vi "TDMS Write.vi"(7 "Channel Name":string, 8 "error in (no error)":errorcluster, 9 "Group Name":string, 10 "TDMS in":refnum<k34>, 11 "I32 in":refnum<class "I32.lvclass">) -> (0 "error out":errorcluster, 2 "TDMS Out":refnum<k34>)   [LabVIEW 2020, in "Data.lvlib" / "I32.lvclass"]
doc: "Write Generic Data to a TDMS file."
uses:
  I32.lvclass
  I32.lvclass/I32.ctl
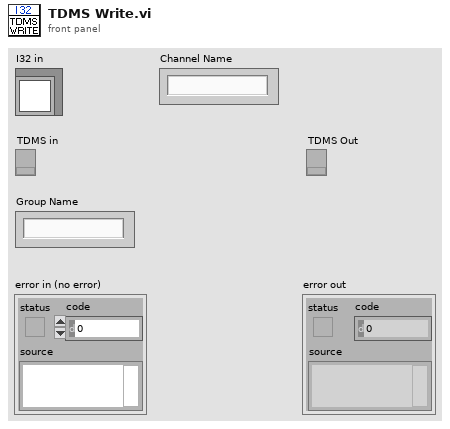
[diagram p1: front panel]
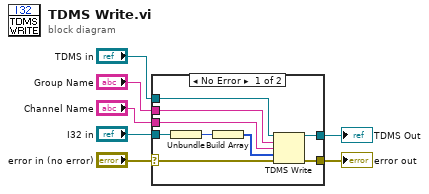
[diagram p0: block diagram]
diagram:
  n1 = case shown="No Error" "error in (no error)" {
    selector: "error in (no error)" -> [w16 w17]
    tunnel: [w15 w17] -> w3
    tunnel: "TDMS in" -> [w14 w18]
    tunnel: [w13 w18] -> w4
    tunnel: "Channel Name" -> [w12 _]
    tunnel: "Group Name" -> [w11 _]
    tunnel: "I32 in" -> [w10 _]
    frame No Error {
      n2 = Unbundle(w10) -> (w9:i32)
      n3 = Build Array(w9) -> (w8:i32[])
      n4 = TDMS Write(0:w14, 5:w11, 7:w12, 9:w8, 11:w16) -> (4:w13:refnum<k34>, 15:w15:errorcluster)  [unwired: 1 in, 2 out]
    }
    frame Error {
    }
  }
  "error out" <- w3
  "TDMS Out" <- w4
